vi "ep_Torque Check Error (N Chan).vi"(0 "phase voltage waveforms":waveform(dbl)[](array[waveform]), 1 "current waveforms":waveform(dbl)[](array[waveform]), 2 "speed in [RPM]":dbl[](array[numeric]), 4 "nameplate information":T1, 5 "error in (no error)":errorcluster, 8 "fundamental frequency [Hz]":dbl=50.0, 9 "total input active power [W]":dbl[](array[numeric]), 10 "reset? (F)":bool, 11 "stator resistance  [ohms]":dbl[](array[numeric])) -> (12 "non-empty speed?":bool, 14 "motor #":i32, 16 "speed out [RPM]":dbl[](array[numeric]), 19 "error out":errorcluster)   [LabVIEW 2014, in "NI_EP_Motor Monitoring.lvlib"]
uses:
  <vilib>/addons/Electrical Power/Motor Monitoring/NI_EP_Motor Monitoring.lvlib
  <vilib>/addons/Electrical Power/Power Measurement/NI_EP_Power Measurement.lvlib
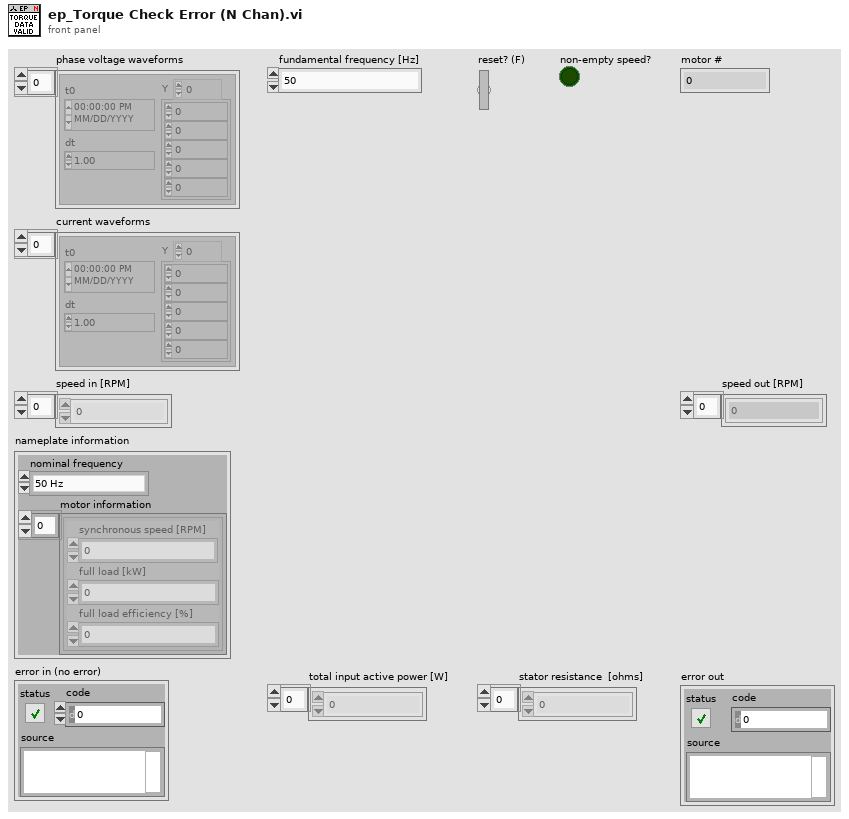
[diagram p1: front panel]
types:
  T1 = cluster{"nominal frequency":enum16{"50 Hz", "60 Hz"}, "motor information":cluster{"synchronous speed [RPM]":dbl, "full load [kW]":dbl, "full load efficiency [%]":dbl}[]}
  T2 = cluster{"synchronous speed [RPM]":dbl, "full load [kW]":dbl, "full load efficiency [%]":dbl}[]
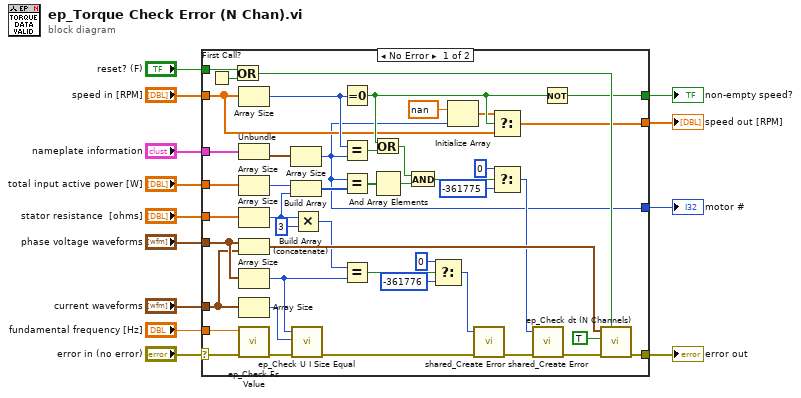
[diagram p0: block diagram]
diagram:
  n1 = case shown="No Error" "error in (no error)" {
    selector: "error in (no error)" -> [w58 w59]
    tunnel: [w38 w59] -> w12
    tunnel: "fundamental frequency [Hz]" -> [w57 _]
    tunnel: "phase voltage waveforms" -> [w56 _]
    tunnel: "current waveforms" -> [w55 _]
    tunnel: "reset? (F)" -> [w52 _]
    tunnel: "total input active power [W]" -> [w49 _]
    tunnel: "stator resistance  [ohms]" -> [w48 _]
    tunnel: "speed in [RPM]" -> [w18 _]
    tunnel: "nameplate information" -> [w47 _]
    tunnel: [w15 _] -> w3
    tunnel: [w14 _] -> w1
    tunnel: [w20 _] -> w2
    frame No Error {
      n2 = First Call?() -> (First Call?: T/F=w53:bool)
      n3 = Or(x=w52, y=w53) -> (x .or. y?=w51:bool)
      n4 = Array Size(array=w18) -> (size(s)=w26:i32)
      n5 = Unbundle(w47) -> ("motor information"=w46:T2)  [unwired: 1 out]
      n6 = Array Size(array=w49) -> (size(s)=w45:i32)
      n7 = Array Size(array=w48) -> (size(s)=w37:i32)
      n8 = Build Array (concatenate)(w56, w55) -> (w54:waveform(dbl)[])
      n9 = Array Size(array=w56) -> (size(s)=w28:i32)
      n10 = Array Size(array=w55) -> (size(s)=w27:i32)
      n11 = call <vilib>:"ep_Check Fs Value.vi"("error in (no error)"=w58, "fundamental frequency [Hz]"=w57) -> ("error out"=w29:errorcluster)  [unwired: 9 in]
      n12 = Array Size(array=w46) -> (size(s)=w15:i32)
      n13 = Build Array(w45, w37) -> (w44:i32[])
      n14 = call <vilib>:"ep_Check U I Size Equal.vi"("error in (no error)"=w29, "current channel number"=w27, "voltage channel number"=w28) -> ("error out"=w21:errorcluster)  [unwired: 8 in]
      n15 = Multiply(x=w37, y=3) -> (x*y=w33:i32)
      n16 = Equal To 0?(x=w26) -> (x = 0?=w19:bool)
      n17 = Equal?(x=w26, y=w15) -> (x = y?=w25:bool)
      n18 = Equal?(x=w15, y=w44) -> (x = y?=w43:bool[])
      n19 = Equal?(x=w33, y=w28) -> (x = y?=w32:bool)
      n20 = Or(x=w19, y=w25) -> (x .or. y?=w24:bool)
      n21 = And Array Elements(Boolean array=w43) -> (logical AND=w23:bool)
      n22 = And(x=w24, y=w23) -> (x .and. y?=w22:bool)
      n23 = Select(t=0, s=w32, f=-361776 ("error code (0)")) -> (s? t:f=w31:i32)
      n24 = Initialize Array(nan, w15) -> (w17:dbl[])
      n25 = call <vilib>:"shared_Create Error.vi"("error in (no error)"=w21, "error code (0)"=w31) -> ("error out"=w40:errorcluster)  [unwired: 9 in]
      n26 = Select(t=w17, s=w19, f=w18) -> (s? t:f=w20:dbl[])
      n27 = Select(t=0, s=w22, f=-361775 ("error code (0)")) -> (s? t:f=w30:i32)
      n28 = call <vilib>:"shared_Create Error.vi"("error in (no error)"=w40, "error code (0)"=w30) -> ("error out"=w39:errorcluster)  [unwired: 9 in]
      n29 = Not(x=w19) -> (.not. x?=w14:bool)
      n30 = call <vilib>:"ep_Check dt (N Channels).vi"("reset? (F)"=w51, "error in (no error)"=w39, "waveforms only? (F)"=TRUE, "waveforms"=w54) -> ("error out"=w38:errorcluster)  [unwired: 3 in, 4 out]
    }
    frame Error {
    }
  }
  "error out" <- w12
  "motor #" <- w3
  "speed out [RPM]" <- w2
  "non-empty speed?" <- w1
